vi "主画面.vi"() -> ()   [LabVIEW 2016]
uses:
  <vilib>/Utility/config.llb/Read Key (String).vi
  <vilib>/Utility/inputDevices.llb/mouseAcquire.vi
  <vilib>/Utility/inputDevices.llb/closeMouse.vi
  <vilib>/Utility/config.llb/NI_LVConfig.lvlib
  data/FreeMem.dll
panel:
  in  "全屏":T1
  out "站点名称":string="站点名称"
  out "时间显示":string="2017-05-09 10:50:42"
  out "Version":string="Version:1.0.0"
  in  "主画面菜单":enum32{"首页", "数据查询", "运维调试", "系统设置"}(xcontrol)
  # "一 体 化 微 型 水 质 监 测 站"
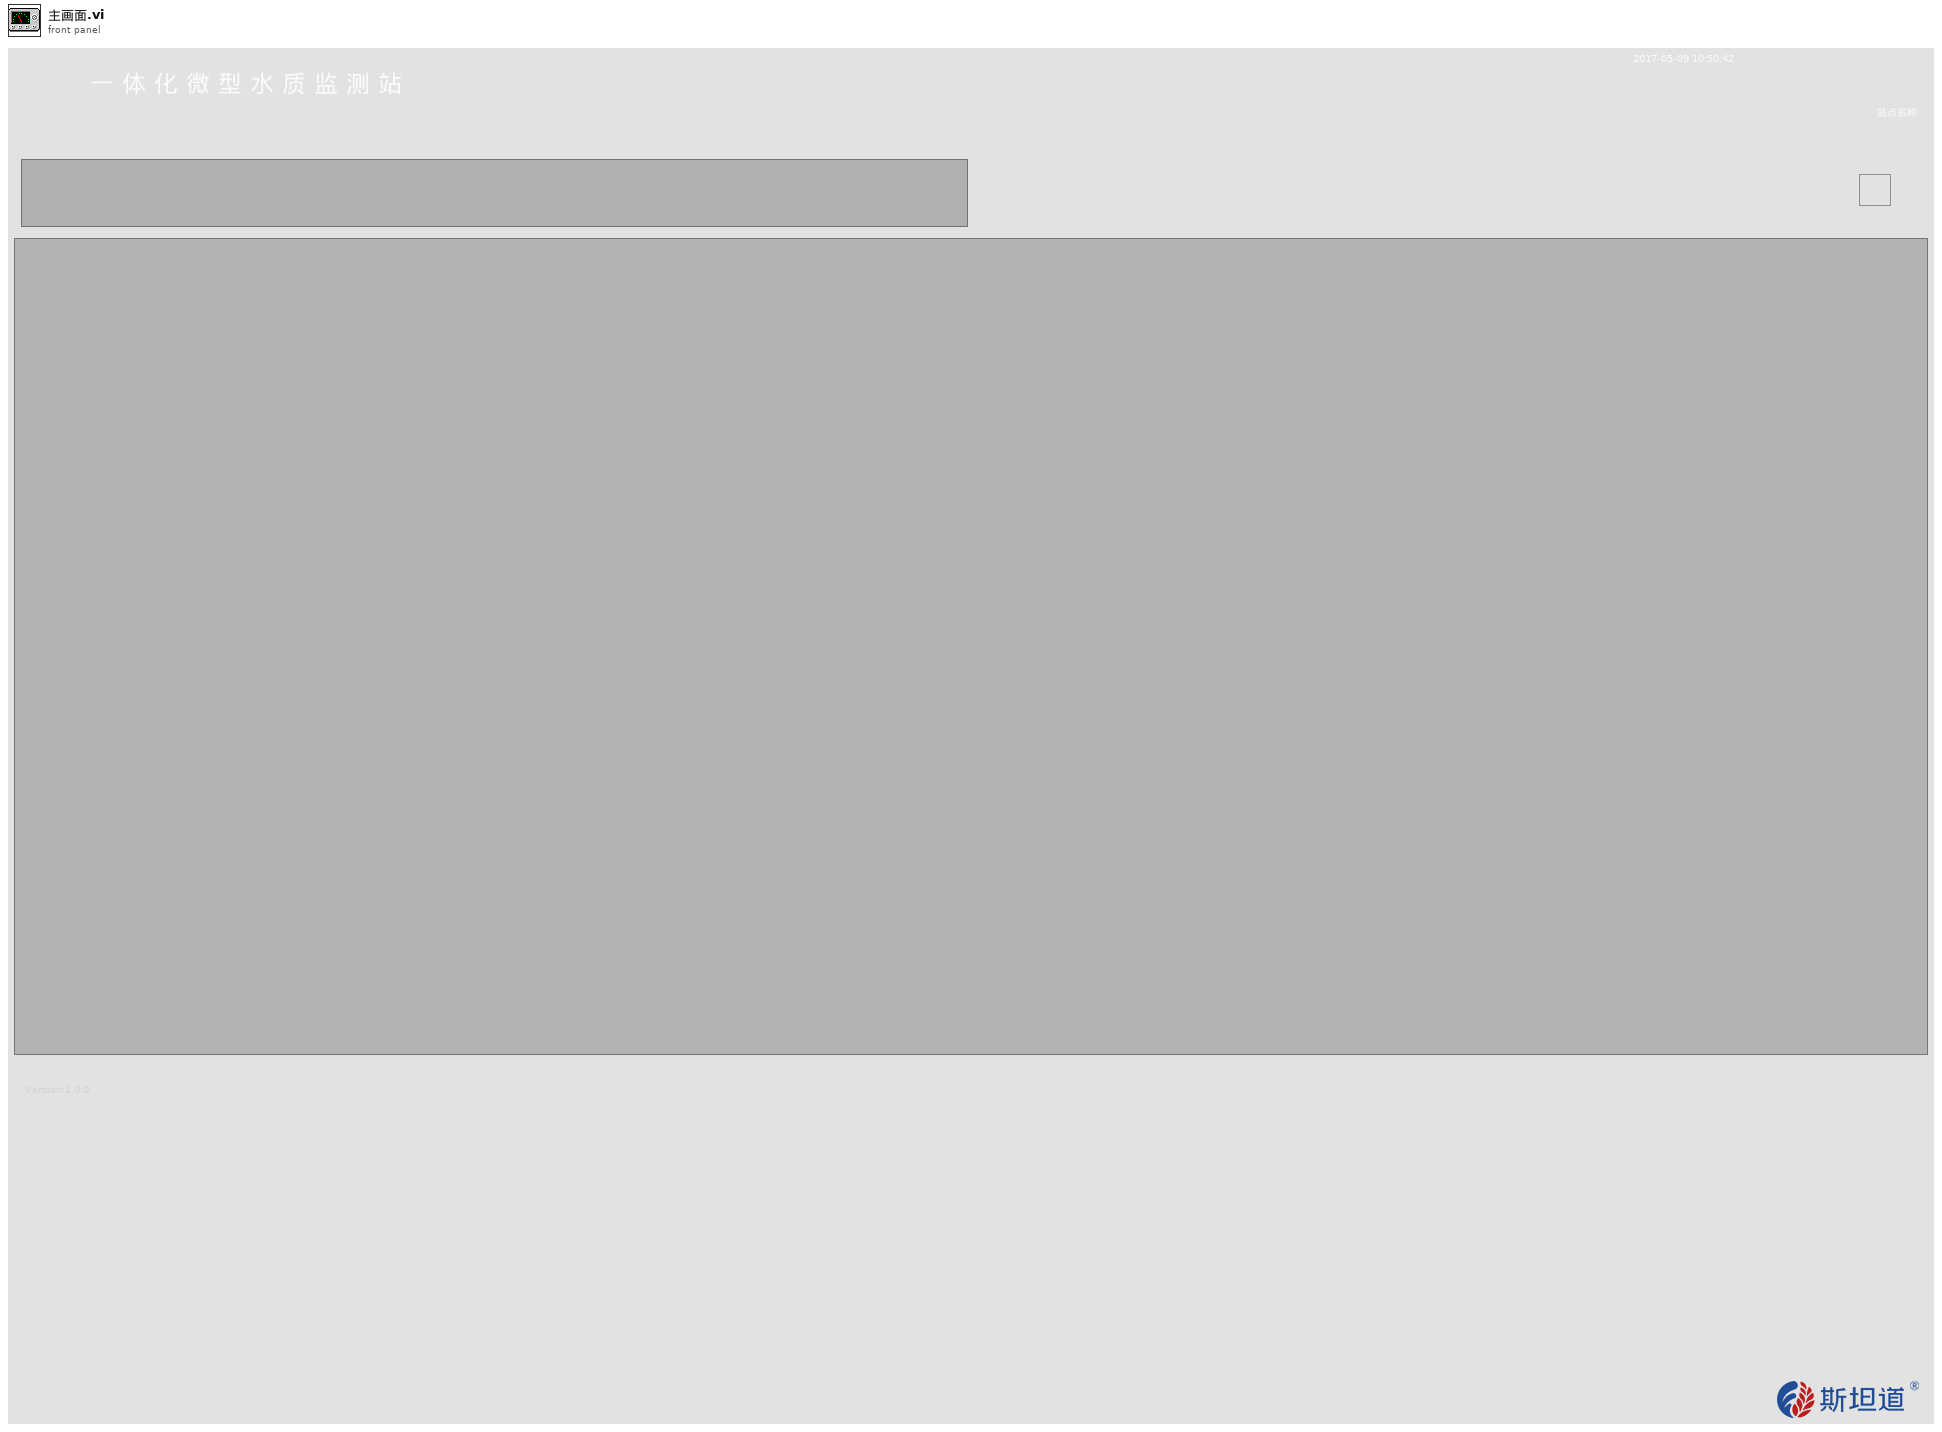
[diagram p1: front panel]
types:
  T1 = typedef "全屏按钮.ctl" = bool
  T2 = cluster{"时间标识":timestamp, "设备":string, "日志信息":string, "流程参数":string}
  T3 = enum32{"invalid app kind", "Development System", "Run Time System", "Student Edition", "Embedded LabVIEW", "Evaluation", "Custom"}
  T4 = typedef "NI_LVConfig.lvlib/Config Data RefNum.ctl" = refnum<k1>
  T5 = cluster{"Horizontal":i32, "Vertical":i32, "Scrolling":i32}
  T6 = enum32{"Bad", "Idle", "Run top level", "Running"}
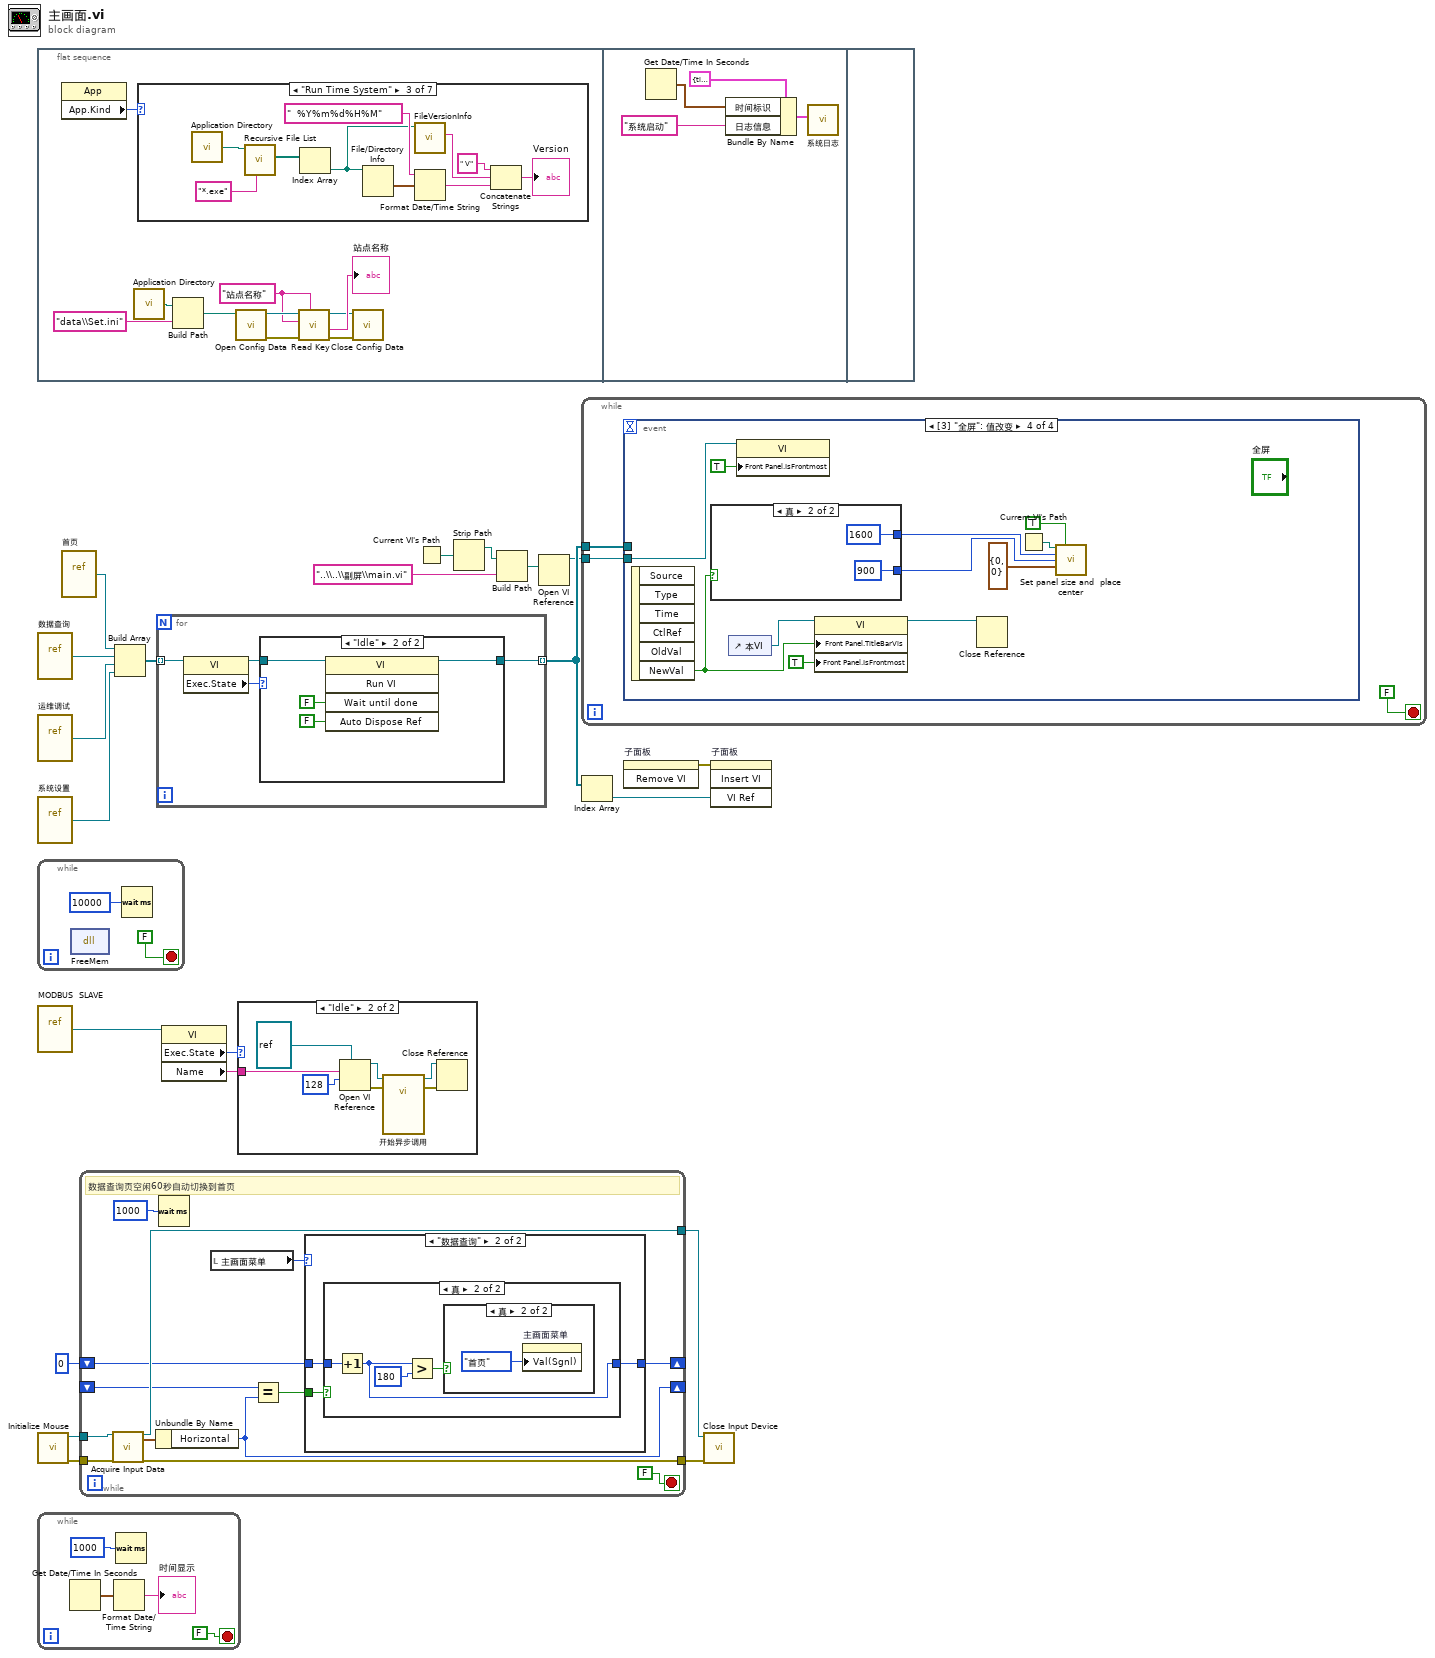
[diagram p0: block diagram]
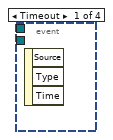
[diagram p13: hidden frame]
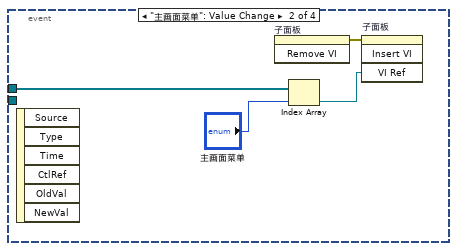
[diagram p14: hidden frame]
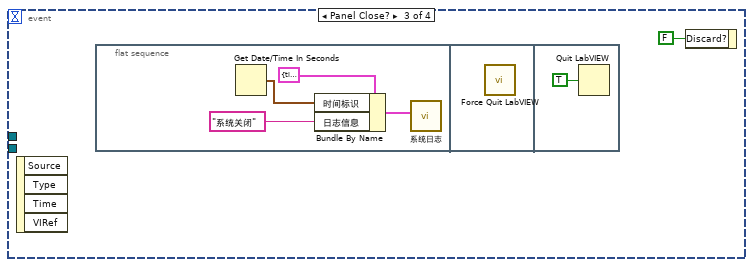
[diagram p15: hidden frame]
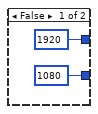
[diagram p16: hidden frame]
diagram:
  n1 = flat-sequence {
    frame #0 {
      w22 = "站点名称" ("section")
      n2 = property class="App"() -> ("App.Kind"=w31:T3)  [unwired: 2 in, 2 out]
      n3 = call <vilib>:"Application Directory.vi"() -> ("Application Directory"=w25:path)
      n4 = case shown="\"Run Time System\"" w31 {
        frame "invalid app kind" {
        }
        frame "Development System", Default {
        }
        frame "Run Time System" {
          n5 = call <vilib>:"Application Directory.vi"() -> ("Application Directory"=w33:path)
          n6 = call <vilib>:"Recursive File List.vi"("pattern"="*.exe", "Folder Path"=w33) -> ("All Files in Dir"=w34:path[])  [unwired: 5 in, 4 out]
          n7 = Index Array(array=w34) -> (element=w32:path)  [unwired: 1 in]
          n8 = File/Directory Info(path=w32) -> (last mod=w38:timestamp)  [unwired: 1 in, 6 out]
          n9 = call <vilib>:"FileVersionInfo.vi"("Application Path in"=w32) -> ("File Version Info"=w40:string)  [unwired: 7 in, 3 out]
          n10 = Format Date/Time String(time format string (%c)="  %Y%m%d%H%M" ("时间格式字符串(%c)"), seconds (now)=w38) -> (date/time string=w36:string)  [unwired: 1 in]
          n11 = Concatenate Strings(" V" ("字符串"), w40, w36) -> (→"Version":string)
        }
        frame "Student Edition" {
        }
        frame "Embedded LabVIEW" {
        }
        frame "Evaluation" {
        }
        frame "Custom" {
        }
      }
      n12 = Build Path(base path=w25, name or relative path="data\\Set.ini" ("名称或相对路径")) -> (appended path=w23:path)
      n13 = call <vilib>:"Open Config Data.vi"("configuration file path"=w23) -> ("error out"=w27:errorcluster, "refnum"=w30:T4)  [unwired: 8 in, 1 out]
      n14 = call-poly <vilib>:"Read Key.vi"("section"=w22, "error in (no error)"=w27, "key"=w22, "refnum"=w30) -> ("error out"=w26:errorcluster, "value"=→"站点名称":string, "refnum out"=w28:T4)  [unwired: 4 in, 1 out]
      n15 = call <vilib>:"Close Config Data.vi"("error in (no error)"=w26, "refnum"=w28) -> ()  [unwired: 8 in, 2 out]
    }
    frame #1 {
      n16 = Get Date/Time In Seconds() -> (seconds since 1Jan1904=w43:timestamp)
      n17 = Bundle By Name(cluster=T2 {"时间标识"=timestamp(0 s since 1904-01-01), "设备"="系统", "日志信息"="", "流程参数"=""} ("data in"), "时间标识"=w43, "日志信息"="系统启动") -> (w44:T2)
      n18 = call "系统日志.vi"("data in"=w44) -> ()  [unwired: 11 in]
    }
    frame #2 {
    }
  }
  n19 = vi-ref "数据查询.vi"() -> (w17:refnum<vi>)
  n20 = vi-ref "运维调试.vi"() -> (w16:refnum<vi>)
  n21 = vi-ref "系统设置.vi"() -> (w15:refnum<vi>)
  n22 = while {
    stop <- FALSE stop-if-true
    n23 = dll-call lib="PTH2iabs CUsersHsiao\tDocumentsGIT一体站模板一体站项目 - 高压过滤dataFreeMem.dll" fn="FreeMem"() -> ()  [unwired: 4 in, 2 out]
    n24 = Wait (ms)(milliseconds to wait=u32 10000 ("等待时间（毫秒）")) -> ()  [unwired: 1 out]
  }
  n25 = vi-ref "MODBUS  SLAVE.vi"() -> (w13:refnum<vi>)
  n26 = call <vilib>:"Initialize Mouse.vi"() -> ("error out"=w4:errorcluster, "device ID"=w5:refnum<k1>)  [unwired: 10 in]
  n27 = while {
    stop <- FALSE stop-if-true
    n28 = Get Date/Time In Seconds() -> (seconds since 1Jan1904=w48:timestamp)
    n29 = Format Date/Time String(seconds (now)=w48) -> (date/time string=→"时间显示":string)  [unwired: 2 in]
    n30 = Wait (ms)(milliseconds to wait=u32 1000 ("等待时间（毫秒）")) -> ()  [unwired: 1 out]
  }
  n31 = vi-ref "首页.vi"() -> (w18:refnum<vi>)
  n32 = while {
    shift-right: [w55] -> _
    shift-left: 0 -> [w56]
    tunnel: w5 -> [w63]
    tunnel: w4 -> [w62]
    tunnel: [w61] -> w3
    tunnel: [w60] -> w2
    shift-right: [w54] -> _
    shift-left: _ -> [w53]
    stop <- FALSE stop-if-true
    # "数据查询页空闲60秒自动切换到首页"
    n33 = call-poly <vilib>:"Acquire Input Data.vi"("device ID"=w63, "error in (no error)"=w62) -> ("device ID"=w61:refnum<k1>, "axis info"=w57:T5, "error out"=w60:errorcluster)  [unwired: 14 in, 1 out]
    n34 = Unbundle By Name(w57) -> ("Horizontal"=w54:i32)
    n35 = Wait (ms)(milliseconds to wait=u32 1000 ("等待时间（毫秒）")) -> ()  [unwired: 1 out]
    n36 = local read "主画面菜单"() -> (w58:enum32{"首页", "数据查询", "运维调试", "系统设置"})
    n37 = Equal?(x=w53, y=w54) -> (x = y?=w52:bool)
    n38 = case shown="\"数据查询\"" w58 {
      tunnel: w56 -> [_ w67]
      tunnel: [_ w66] -> w55
      tunnel: w52 -> [_ w65]
      frame "首页", Default {
      }
      frame "数据查询" {
        n39 = case shown="真" w65 {
          tunnel: w67 -> [_ w71]
          tunnel: [_ w70] -> w66
          frame False {
          }
          frame True {
            n40 = Increment(x=w71) -> (x+1=w70:i32)
            n41 = Greater?(x=w70, y=180) -> (0:w68:bool)
            n42 = case shown="真" w68 {
              frame False {
              }
              frame True {
                n43 = property on="主画面菜单" class="主画面菜单 (严格)"("Val(Sgnl)"=enum32{"首页", "数据查询", "运维调试", "系统设置"}."首页" ("值(信号)")) -> ()  [unwired: 2 in, 2 out]
              }
            }
          }
        }
      }
    }
  }
  n44 = Build Array(w18, w17, w16, w15) -> (w14:refnum<vi>[])
  n45 = for {
    tunnel: w14 -> [w76] mode=indexing
    tunnel: [w73] -> w20 mode=indexing
    n46 = property class="VI"(reference=w76) -> (reference out=w74:refnum<vi>, "Exec.State"=w75:T6)  [unwired: 1 in, 1 out]
    n47 = case shown="\"Idle\"" w75 {
      tunnel: w74 -> [w77 w79]
      tunnel: [w77 w78] -> w73
      frame "Bad", Default {
      }
      frame "Idle" {
        n48 = invoke class="VI" method="Run VI"(reference=w79, "Wait until done"=FALSE ("结束前等待"), "Auto Dispose Ref"=FALSE ("自动销毁引用")) -> (reference out=w78:refnum<vi>)  [unwired: 2 in, 4 out]
      }
    }
  }
  n49 = property class="VI"(reference=w13) -> ("Exec.State"=w12:T6, "Name"=w11:string)  [unwired: 1 in, 2 out]
  n50 = case shown="\"Idle\"" w12 {
    tunnel: w11 -> [_ w82]
    frame "Bad", Default {
    }
    frame "Idle" {
      n51 = Open VI Reference(type specifier VI Refnum (for type only)=refnum<vi> refnum, vi path=w82, options=128 ("选项")) -> (vi reference=w84:refnum<vi>, error out=w87:errorcluster)  [unwired: 3 in]
      n52 = call-by-ref "开始异步调用"(reference=w84, error in=w87) -> (reference out=w86:refnum<vi>, error out=w88:errorcluster)  [unwired: 11 in, 1 out]
      n53 = Close Reference(reference=w86, error in (no error)=w88) -> ()  [unwired: 1 out]
    }
  }
  n54 = Current VI's Path() -> (path=w10:path)
  n55 = Strip Path(path=w10) -> (stripped path=w9:path)  [unwired: 1 out]
  n56 = Build Path(base path=w9, name or relative path="..\\..\\副屏\\main.vi" ("名称或相对路径")) -> (appended path=w7:path)
  n57 = Open VI Reference(vi path=w7) -> (vi reference=w6:refnum<vi>)  [unwired: 5 in, 1 out]
  n58 = while {
    tunnel: w20 -> [w90]
    tunnel: w6 -> [w89]
    stop <- FALSE stop-if-true
    n59 = event shown="[3] \"全屏\": 值改变" {
      selector: _ -> [_ _ _ _]
      dyn-events: _ -> [_ _ _ _]
      timeout: _ -> [_ _ _ _]
      tunnel: w90 -> [_ w94 _ _]
      tunnel: w89 -> [_ _ _ w103]
      event Timeout {
        n60 = event-data() -> ()  [unwired: 1 in, 3 out]
      }
      event "主画面菜单": Value Change {
        n61 = event-data() -> ()  [unwired: 1 in, 6 out]
        n62 = invoke on="子面板" class="SubPnl" method="Remove VI"() -> (error out=w92:errorcluster)  [unwired: 3 in, 2 out]
        n63 = Index Array(array=w94, index="主画面菜单") -> (element=w93:refnum<vi>)
        n64 = invoke on="子面板" class="SubPnl" method="Insert VI"(error in=w92, "VI Ref"=w93) -> ()  [unwired: 2 in, 4 out]
      }
      event Panel Close? {
        n65 = event-data() -> ()  [unwired: 1 in, 4 out]
        n66 = flat-sequence {
          frame #0 {
            n67 = Get Date/Time In Seconds() -> (seconds since 1Jan1904=w99:timestamp)
            n68 = Bundle By Name(cluster=T2 {"时间标识"=timestamp(0 s since 1904-01-01), "设备"="系统", "日志信息"="", "流程参数"=""} ("data in"), "时间标识"=w99, "日志信息"="系统关闭") -> (w98:T2)
            n69 = call "系统日志.vi"("data in"=w98) -> ()  [unwired: 11 in]
          }
          frame #1 {
            n70 = call "Force Quit LabVIEW.vi"() -> ()  [unwired: 10 in, 2 out]
          }
          frame #2 {
            n71 = Quit LabVIEW(quit? (T)=TRUE ("退出？(T)")) -> ()
          }
        }
        n72 = event-data("Discard?"=FALSE ("放弃？")) -> ()  [unwired: 1 in, 1 out]
      }
      event Value Change {
        n73 = event-data() -> ("NewVal"=w107:T1)  [unwired: 1 in, 5 out]
        n74 = case shown="真" w107 {
          tunnel: [1920 ("Panel Width") 1600 ("Panel Width")] -> w106
          tunnel: [1080 ("Panel Height") 900 ("Panel Height")] -> w105
          frame False {
          }
          frame True {
          }
        }
        n75 = control-ref of="本VI"() -> (w112:refnum<vi>)
        n76 = property class="VI"(reference=w103, "Front Panel.IsFrontmost"=TRUE ("前面板窗口:在最前")) -> ()  [unwired: 1 in, 2 out]
        n77 = property class="VI"(reference=w112, "Front Panel.TitleBarVis"=w107, "Front Panel.IsFrontmost"=TRUE ("前面板窗口:在最前")) -> (reference out=w108:refnum<vi>)  [unwired: 1 in, 1 out]
        n78 = Close Reference(reference=w108) -> ()  [unwired: 1 in, 1 out]
        n79 = Current VI's Path() -> (path=w111:path)
        n80 = call "Set panel size and  place center.vi"("Path"=w111, "Close Reference (false)"=TRUE, "Panel Width"=w106, "Panel Height"=w105, "FP.Origin in(H & V)"=cluster{"Horizontal":i16, "Vertical":i16} {"Horizontal"=0, "Vertical"=0}) -> ()  [unwired: 6 in, 5 out]
      }
    }
  }
  n81 = Index Array(array=w20) -> (element=w19:refnum<vi>)  [unwired: 1 in]
  n82 = invoke on="子面板" class="SubPnl" method="Remove VI"() -> (error out=w21:errorcluster)  [unwired: 3 in, 2 out]
  n83 = call-poly <vilib>:"Close Input Device.vi"("error in (no error)"=w2, "device ID"=w3) -> ()  [unwired: 8 in, 1 out]
  n84 = invoke on="子面板" class="SubPnl" method="Insert VI"(error in=w21, "VI Ref"=w19) -> ()  [unwired: 2 in, 4 out]
